vi "DHE_custom.vi"(0 "fd":i32, 7 "args":string, 11 "error in (no error)":errorcluster) -> (4 "fd out":i32, 8 "str result":string, 15 "error out":errorcluster)   [LabVIEW 2016]
doc: "This VI closes the I/O interface with the instrument."
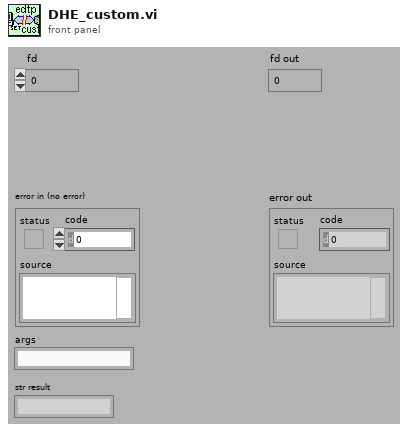
[diagram p1: front panel]
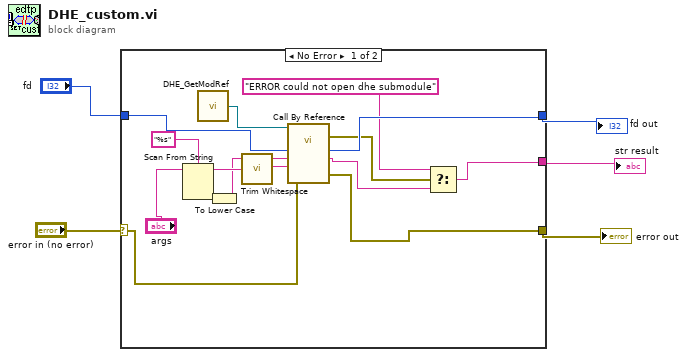
[diagram p0: block diagram]
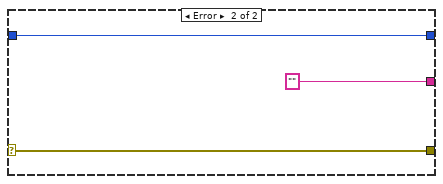
[diagram p2: hidden frame]
diagram:
  n1 = case shown="No Error" "error in (no error)" {
    selector: "error in (no error)" -> [w17 w22]
    tunnel: "fd" -> [w18 w23]
    tunnel: [w10 w22] -> w4
    tunnel: [w19 w23] -> w3
    tunnel: [w7 "" ("str result")] -> w1
    frame No Error {
      n2 = Scan From String(format string="%s", input string="args") -> (remaining string=w13:string, output 1=w14:string)  [unwired: 2 in, 3 out]
      n3 = call "DHE_GetModRef.vi"() -> ("DHE_ModRef"=w20:refnum<vi>)  [unwired: 9 out]
      n4 = To Lower Case(string=w14) -> (all lower case string=w12:string)
      n5 = call <vilib>:"Trim Whitespace.vi"("string"=w13) -> ("trimmed string"=w11:string)  [unwired: 1 in]
      n6 = call-by-ref "?"(reference=w20, "error in (no error)"=w17, "arguments"=w11, "function"=w12, "fd in"=w18) -> (error out=w9:errorcluster, 0:"error out"=w10:errorcluster, "str result"=w8:string, "fd out"=w19:i32)  [unwired: 5 in, 2 out]
      n7 = Select(t="ERROR could not open dhe submodule", s=w9, f=w8) -> (s? t:f=w7:string)
    }
    frame Error {
    }
  }
  "error out" <- w4
  "fd out" <- w3
  "str result" <- w1
